vi "Check for Pres Sensor Cali (SH).vi"(8 "error in (no error)":errorcluster, 9 "Intercept in":dbl, 10 "Slope in":dbl, 11 "Boolean":bool) -> (0 "error out":errorcluster, 2 "Intercept out":dbl, 3 "Slope out":dbl)   [LabVIEW 2013]
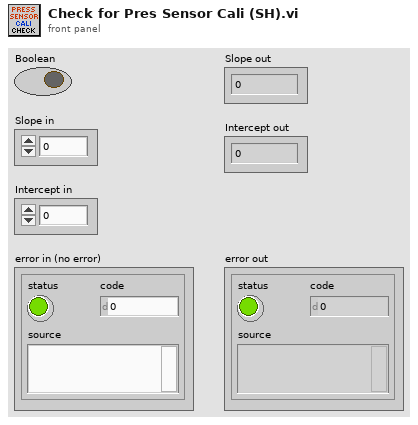
[diagram p1: front panel]
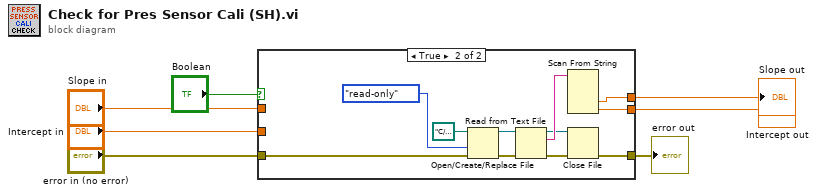
[diagram p0: block diagram]
diagram:
  n1 = case shown="True" "Boolean" {
    tunnel: "Intercept in" -> [w10 _]
    tunnel: [w10 w21] -> w6
    tunnel: "Slope in" -> [w9 _]
    tunnel: [w9 w20] -> w7
    tunnel: "error in (no error)" -> [w8 w19]
    tunnel: [w8 w18] -> w2
    frame False {
    }
    frame True {
      n2 = Open/Create/Replace File(file path (use dialog)=path "C:/Users/scholp/Desktop/Calibration .txt files/SH Pressure Cali.txt", error in=w19, access (0:read/write)=enum16{"read/write", "read-only", "write-only"}."read-only") -> (refnum out=w14:refnum<file>, error out=w16:errorcluster)  [unwired: 3 in, 1 out]
      n3 = Read from Text File(file (use dialog)=w14, error in=w16) -> (refnum out=w13:refnum<file>, text=w15:string, error out=w17:errorcluster)  [unwired: 2 in, 1 out]
      n4 = Scan From String(input string=w15) -> (output 1=w20:dbl, output 2=w21:dbl)  [unwired: 5 in, 3 out]
      n5 = Close File(refnum=w13, error in=w17) -> (error out=w18:errorcluster)  [unwired: 1 out]
    }
  }
  "Slope out" <- w7
  "Intercept out" <- w6
  "error out" <- w2
